vi "AVPP_Destructor.vi"(8 "error in (no error)":errorcluster, 10 "AVPP class":refnum<data-value>, 11 "AVPP in":refnum<class "AVPP.lvclass">) -> (0 "error out":errorcluster, 3 "AVPP out":refnum<class "AVPP.lvclass">)   [LabVIEW 2014, in "AVPP.lvclass"]
doc: "Close AVPP class"
uses:
  AVPP.lvclass
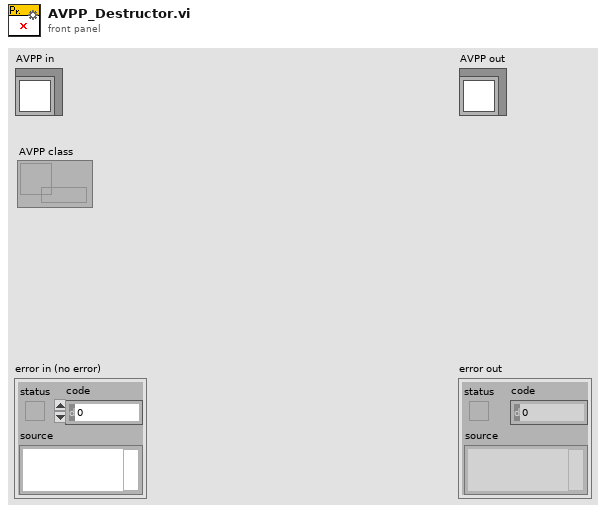
[diagram p1: front panel]
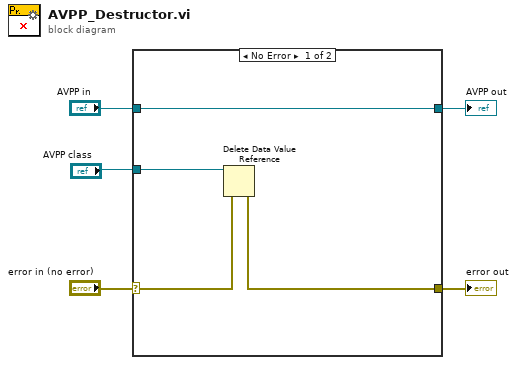
[diagram p0: block diagram]
diagram:
  n1 = case shown="No Error" "error in (no error)" {
    selector: "error in (no error)" -> [w8 w11]
    tunnel: [w7 w11] -> w4
    tunnel: [w6 w10] -> w2
    tunnel: "AVPP in" -> [w6 w10]
    tunnel: "AVPP class" -> [w9 _]
    frame No Error {
      n2 = Delete Data Value Reference(data value reference=w9, error in=w8) -> (error out=w7:errorcluster)  [unwired: 1 out]
    }
    frame Error {
    }
  }
  "error out" <- w4
  "AVPP out" <- w2
